vi "Get VI Ref.vi"(8 "error in":errorcluster, 11 "Class in":refnum<class>) -> (0 "error out":errorcluster, 2 "VI Refnum":refnum<vi>, 3 "Class out":refnum<class>)   [LabVIEW 2023, in "Label-Driven UI.lvlib"]
doc: "클래스에 매칭된 VI 참조를 얻습니다."
uses:
  Label-Driven UI.lvlib
  Map Cmd.ctl
  <vilib>/Utility/error.llb/Error Cluster From Error Code.vi
  <vilib>/ErrorRing/Error Ring.xnode
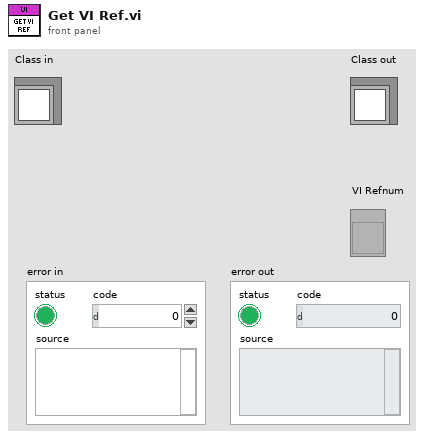
[diagram p1: front panel]
types:
  T1 = typedef "Label-Driven UI.lvlib/Map Cmd.ctl" = enum16{"Insert", "Delete", "Look"}
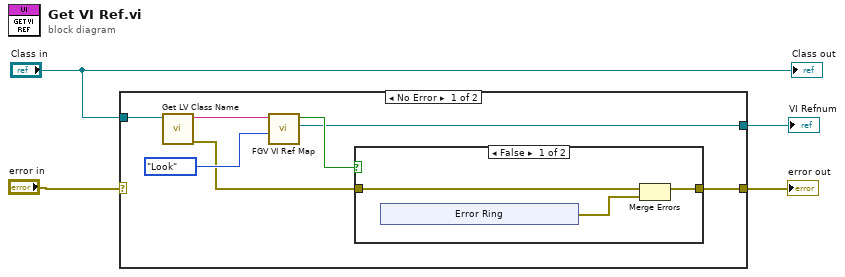
[diagram p0: block diagram]
diagram:
  n1 = case shown="No Error" "error in" {
    selector: "error in" -> [_ w21]
    tunnel: [w9 w21] -> w1
    tunnel: [w8 _] -> w3
    tunnel: "Class in" -> [w7 _]
    frame No Error {
      n2 = call <vilib>:"Get LV Class Name.vi"("object"=w7) -> ("error out"=w5:errorcluster, "class name"=w6:string)  [unwired: 9 in]
      n3 = call "FGV VI Ref Map.vi"("Map Cmd"=Map_Cmd."Look", "Class Name"=w6) -> ("VI Ref out"=w8:refnum<vi>, "isExist"=w10:bool)  [unwired: 8 in]
      n4 = case shown="False" w10 {
        tunnel: w5 -> [w13 w20]
        tunnel: [w12 w20] -> w9
        frame False {
          n5 = xnode "Error Ring"() -> ("error out"=w14:errorcluster)
          n6 = Merge Errors(w13, w14) -> (w12:errorcluster)
        }
        frame True {
        }
      }
    }
    frame Error {
    }
  }
  "VI Refnum" <- w3
  "error out" <- w1
  "Class out" <- "Class in"
